vi "Get Folder Names.vi"(11 "Parent Tag":string) -> (3 "Folder Names":string[](array[string]))   [LabVIEW 2019, in "Tree Browser.lvlib"]
doc: "Gets the folder listing for a given parent tag (parent path). If parent tag is _ROOT_, returns a list of available disks (C:\\, D:\\, etc)."
uses:
  Tree Browser.lvlib
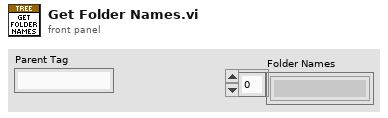
[diagram p1: front panel]
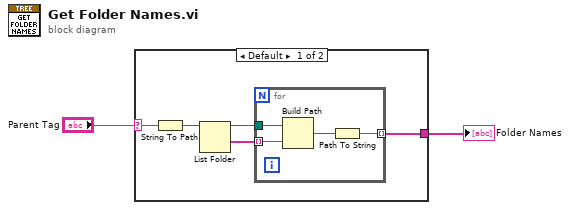
[diagram p0: block diagram]
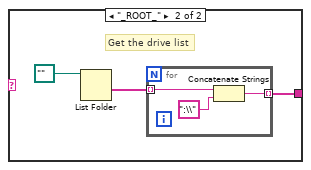
[diagram p2: hidden frame]
diagram:
  n1 = case shown="Default" "Parent Tag" {
    selector: "Parent Tag" -> [w7 _]
    tunnel: [w3 w12] -> w1
    frame Default {
      n2 = String To Path(string=w7) -> (path=w6:path)
      n3 = List Folder(path=w6) -> (path out=w4:path, folder names=w5:string[])  [unwired: 3 in, 2 out]
      n4 = for {
        tunnel: w5 -> [w11] mode=indexing
        tunnel: w4 -> [w10]
        tunnel: [w8] -> w3 mode=indexing
        n5 = Build Path(base path=w10, name or relative path=w11) -> (appended path=w9:path)
        n6 = Path To String(path=w9) -> (string=w8:string)
      }
    }
    frame "_ROOT_" {
      # "Get the drive list"
      n7 = List Folder(path=path "") -> (folder names=w13:string[])  [unwired: 3 in, 3 out]
      n8 = for {
        tunnel: w13 -> [w16] mode=indexing
        tunnel: [w15] -> w12 mode=indexing
        n9 = Concatenate Strings(w16, ":\\" ("string")) -> (w15:string)
      }
    }
  }
  "Folder Names" <- w1
